vi "Write Relative Folder Path.vi"(8 "error in":errorcluster, 10 "Relative Folder Path":path=path "approvals", 11 "Namer with Folder in":refnum<class "Namer with Folder.lvclass">) -> (0 "error out":errorcluster, 3 "Namer with Folder out":refnum<class "Namer with Folder.lvclass">)   [LabVIEW 2026, in "Approval Tests.lvlib" / "Namer with Folder.lvclass"]
uses:
  Namer with Folder.lvclass
  Namer with Folder.lvclass/Namer with Folder.ctl
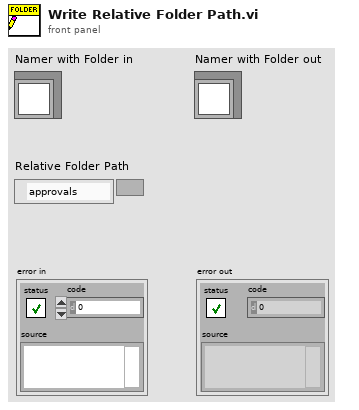
[diagram p1: front panel]
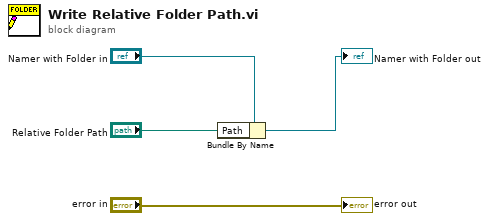
[diagram p0: block diagram]
diagram:
  n1 = Bundle By Name(cluster="Namer with Folder in", "Path"="Relative Folder Path") -> (→"Namer with Folder out":refnum<class "Namer with Folder.lvclass">)
  "error out" <- "error in"
